vi "Update Controller State.vi"(8 "error in (no error)":errorcluster, 11 "Elevator Controller Actor in":refnum<class "Elevator Controller Actor.lvclass">) -> (0 "error out":errorcluster, 3 "Elevator Controller Actor out":refnum<class "Elevator Controller Actor.lvclass">)   [LabVIEW 2022 SP3, in "Elevator Controller Actor.lvlib" / "Elevator Controller Actor.lvclass"]
uses:
  Elevator Controller Actor.lvclass
  C:/Program Files/National Instruments/LabVIEW 2022/vi.lib/ActorFramework/Actor/Actor.lvclass
  <vilib>/ActorFramework/Actor/Actor.lvclass/Actor.ctl
  <vilib>/ActorFramework/Message Enqueuer/Message Enqueuer.lvclass/Message Enqueuer.ctl
  Elevator Controller Actor.lvclass/Elevator Controller Actor.ctl
  Sim User Console Actor/Elevator Controller Actor/Floor Selection.ctl
  Sim User Console Actor/Elevator Controller Actor/Elevator Call.ctl
  Sim User Console Actor/Elevator Controller Actor/Door Buttons.ctl
  Sim Display Console Actor/Elevator Controller Actor/Elevator Direction.ctl
  Sim Display Console Actor/Elevator Controller Actor/Floor -Enum.ctl
  Configuration Database Actor/Configuration Database Actor/Record -Cluster.ctl
  Configuration Database Actor/Configuration Database Actor Messages/Write Record Msg/Write Record Msg.lvclass/Write Record Msg.ctl
  Sim Sensor Interface Actor/Sim Sensor Interface Actor Messages/Update Elevator Position Msg/Update Elevator Position Msg.lvclass/Update Elevator Position Msg.ctl
  Sim Display Console Actor/Sim Display Console Actor Messages/Update Door Open Msg/Update Door Open Msg.lvclass/Update Door Open Msg.ctl
  Sim Display Console Actor/Sim Display Console Actor Messages/Update Elevator Direction Msg/Update Elevator Direction Msg.lvclass/Update Elevator Direction Msg.ctl
  Sim Display Console Actor/Sim Display Console Actor Messages/Update Elevator Location Msg/Update Elevator Location Msg.lvclass/Update Elevator Location Msg.ctl
  Sim Display Console Actor/Sim Display Console Actor Messages/Update Emergency Msg/Update Emergency Msg.lvclass/Update Emergency Msg.ctl
  Sim Display Console Actor/Sim Display Console Actor Messages/Update Timing Msg/Update Timing Msg.lvclass/Update Timing Msg.ctl
  Sim User Console Actor/Sim User Console Actor Messages/Update Door Buttons Msg/Update Door Buttons Msg.lvclass/Update Door Buttons Msg.ctl
  Sim User Console Actor/Sim User Console Actor Messages/Update Elevator Call Msg/Update Elevator Call Msg.lvclass/Update Elevator Call Msg.ctl
  Sim User Console Actor/Sim User Console Actor Messages/Update Emergency Msg/Update Emergency Msg.lvclass/Update Emergency Msg.ctl
  Sim User Console Actor/Sim User Console Actor Messages/Update Foor Selection Msg/Update Foor Selection Msg.lvclass/Update Foor Selection Msg.ctl
  <vilib>/ActorFramework/Message Enqueuer/Init from Existing Queue.vi
  <vilib>/ActorFramework/Message Enqueuer/Enqueue.vi
  Configuration Database Actor/Configuration Database Actor Messages/Read Record Msg/Read Record Msg.lvclass
  C:/Program Files/National Instruments/LabVIEW 2022/vi.lib/ActorFramework/Message/Message.lvclass
  Configuration Database Actor/Configuration Database Actor Messages/Write Record Msg/Write Record Msg.lvclass
  Sim Sensor Interface Actor/Sim Sensor Interface Actor Messages/Update Elevator Position Msg/Update Elevator Position Msg.lvclass
  Sim Display Console Actor/Sim Display Console Actor Messages/Update Door Open Msg/Update Door Open Msg.lvclass
  Sim Display Console Actor/Sim Display Console Actor Messages/Update Elevator Direction Msg/Update Elevator Direction Msg.lvclass
  Sim Display Console Actor/Sim Display Console Actor Messages/Update Elevator Location Msg/Update Elevator Location Msg.lvclass
  Sim Display Console Actor/Sim Display Console Actor Messages/Update Emergency Msg/Update Emergency Msg.lvclass
  Sim Display Console Actor/Sim Display Console Actor Messages/Update Timing Msg/Update Timing Msg.lvclass
  Sim User Console Actor/Sim User Console Actor Messages/Update Door Buttons Msg/Update Door Buttons Msg.lvclass
  Sim User Console Actor/Sim User Console Actor Messages/Update Elevator Call Msg/Update Elevator Call Msg.lvclass
  Sim User Console Actor/Sim User Console Actor Messages/Update Emergency Msg/Update Emergency Msg.lvclass
  Sim User Console Actor/Sim User Console Actor Messages/Update Foor Selection Msg/Update Foor Selection Msg.lvclass
  Sim User Console Actor/Sim User Console Actor Messages/Read Elevator Call and Floor Selection Msg/Read Elevator Call and Floor Selection Msg.lvclass
  <vilib>/ActorFramework/Message Priority Queue/Priority Enqueue.vi
  <vilib>/ActorFramework/Message Enqueuer/Message Enqueuer.lvclass
  Configuration Database Actor/Configuration Database Actor/Configuration Database Actor.lvclass
  Sim User Console Actor/Elevator Controller Actor/Sim User Console Actor.lvclass
  <vilib>/ActorFramework/Actor/Actor.lvclass
  Sim Display Console Actor/Elevator Controller Actor/Sim Display Console Actor.lvclass
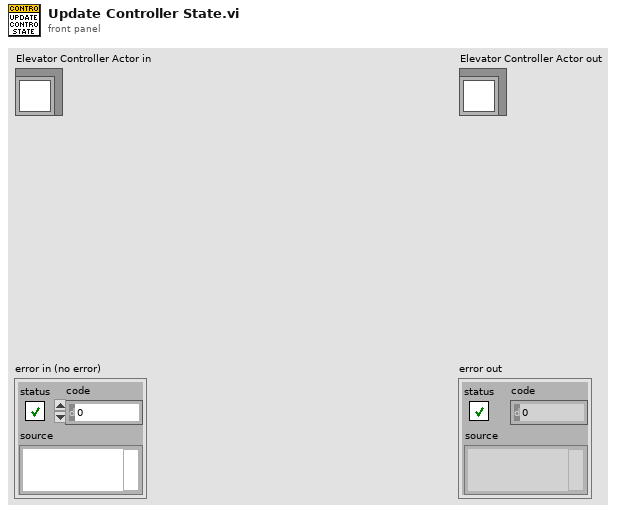
[diagram p1: front panel]
types:
  T1 = typedef "Sim Display Console Actor.lvlib/Sim Display Console Actor.lvclass/Floor -Enum.ctl" = enum16{"1st", "2nd", "3rd", "4th"}
  T2 = typedef "Sim Display Console Actor.lvlib/Sim Display Console Actor.lvclass/Elevator Direction.ctl" = cluster{"Up":bool, "Down":bool}
  T3 = typedef "Sim User Console Actor.lvlib/Sim User Console Actor.lvclass/Door Buttons.ctl" = cluster{"Open Door":bool, "Close Door":bool}
  T4 = typedef "Sim User Console Actor.lvlib/Sim User Console Actor.lvclass/Elevator Call.ctl" = cluster{"Up":bool, "Up 2":bool, "Up 3":bool, "Down":bool, "Down 2":bool, "Down 3":bool}
  T5 = typedef "Sim User Console Actor.lvlib/Sim User Console Actor.lvclass/Floor Selection.ctl" = cluster{"Floor4":bool, "Floor 3":bool, "Floor2":bool, "Floor1":bool}
  T6 = typedef "Configuration Database Actor.lvlib/Configuration Database Actor.lvclass/Record -Cluster.ctl" = cluster{"Door Open":dbl, "Door Close":dbl, "Travel Time":dbl, "Inactivity Time":dbl}
  T7 = typedef "Elevator Controller Actor.lvlib/Elevator Controller Actor.lvclass/State -Enum.ctl" = enum16{"Initial", "Wait for First Request", "Start and Move", "Anaysis", "Continue Travel", "Stop at Floor", "Open and Close Door Sequence", "No Request Remaining", "Emergency Call", "Terminate Process"}
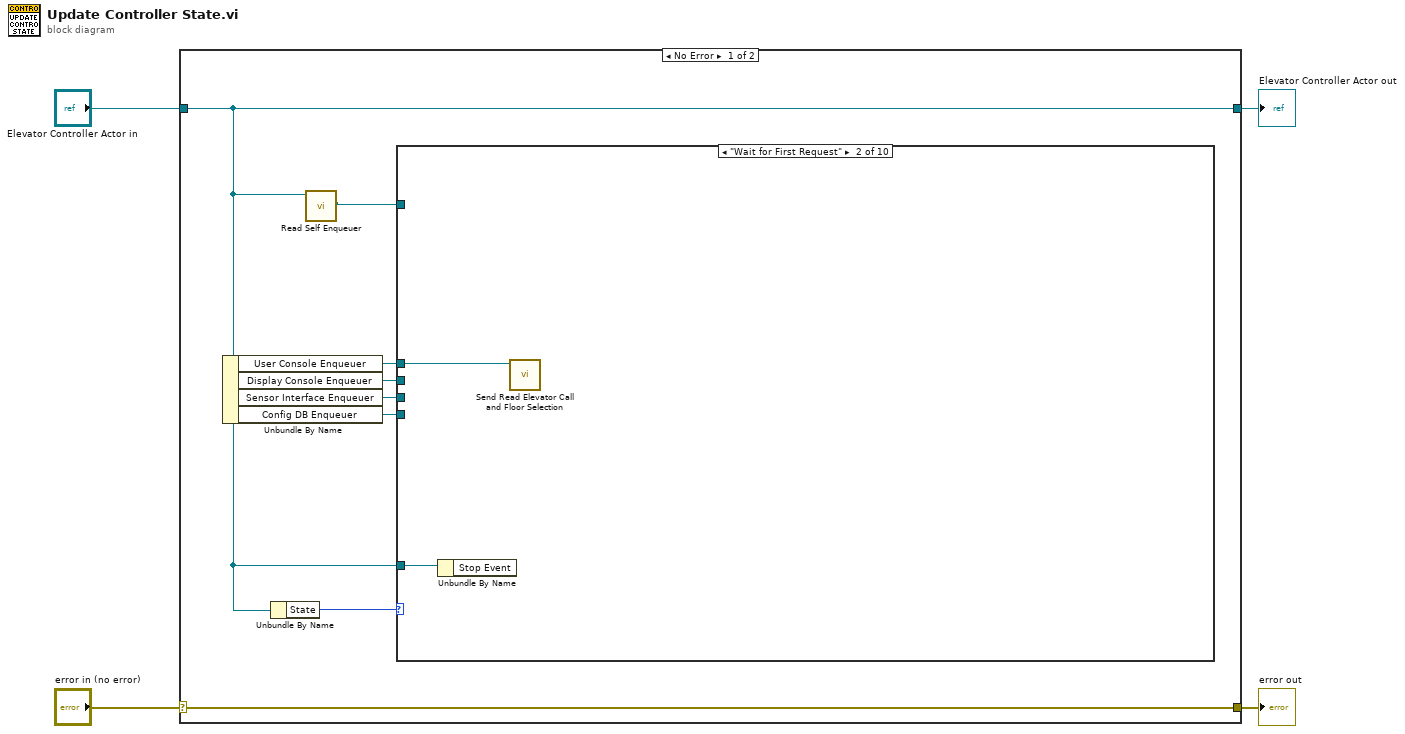
[diagram p0: block diagram]
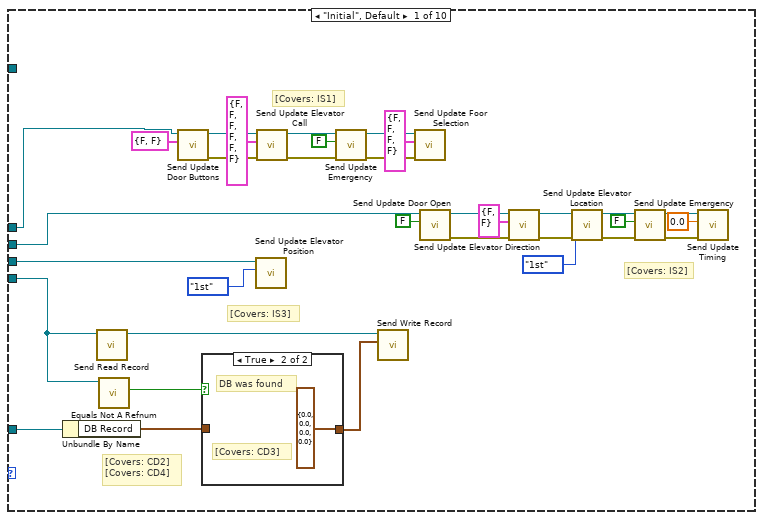
[diagram p2: hidden frame]
diagram:
  n1 = case shown="No Error" "error in (no error)" {
    selector: "error in (no error)" -> [w12 w51]
    tunnel: [w12 w51] -> w3
    tunnel: [w6 w50] -> w1
    tunnel: "Elevator Controller Actor in" -> [w6 w50]
    frame No Error {
      n2 = Unbundle By Name(w6) -> ("User Console Enqueuer"=w10:refnum<class "Message Enqueuer.lvclass">, "Display Console Enqueuer"=w9:refnum<class "Message Enqueuer.lvclass">, "Sensor Interface Enqueuer"=w8:refnum<class "Message Enqueuer.lvclass">, "Config DB Enqueuer"=w7:refnum<class "Message Enqueuer.lvclass">)
      n3 = Unbundle By Name(w6) -> ("State"=w11:T7)
      n4 = call <vilib>:"Read Self Enqueuer.vi"("Actor"=w6) -> ("Self Enqueuer"=w5:refnum<class "Message Enqueuer.lvclass">)  [unwired: 10 in]
      n5 = case shown="\"Wait for First Request\"" w11 {
        tunnel: w10 -> [w29 w49 _ _ _ _ _ _ _ _]
        tunnel: w9 -> [w20 _ _ _ _ _ _ _ _ _]
        tunnel: w8 -> [w14 _ _ _ _ _ _ _ _ _]
        tunnel: w7 -> [w43 _ _ _ _ _ _ _ _ _]
        tunnel: w6 -> [w44 w48 _ _ _ _ _ _ _ _]
        tunnel: w5 -> [_ _ _ _ _ _ _ _ _ _]
        frame "Initial", Default {
          # "[Covers: IS3]"
          # "[Covers: IS2]"
          # "[Covers: IS1]"
          # "[Covers: CD2] \n[Covers: CD4]"
          n6 = Unbundle By Name(w44) -> ("DB Record"=w41:T6)
          n7 = call "Send Read Record.vi"("Message Enqueuer"=w43) -> ("Message Enqueuer out"=w45:refnum<class "Message Enqueuer.lvclass">)  [unwired: 9 in, 1 out]
          n8 = call <vilib>:"Equals Not A Refnum.vi"("Message Enqueuer"=w43) -> ("Not a refnum?"=w42:bool)  [unwired: 10 in]
          n9 = call "Send Update Door Buttons.vi"("Door Buttons"=T3 {"Open Door"=FALSE, "Close Door"=FALSE}, "Message Enqueuer"=w29) -> ("error out"=w39:errorcluster, "Message Enqueuer out"=w36:refnum<class "Message Enqueuer.lvclass">)  [unwired: 8 in]
          n10 = case shown="True" w42 {
            tunnel: w41 -> [w46 _]
            tunnel: [w46 T6 {"Door Open"=0.0, "Door Close"=0.0, "Travel Time"=0.0, "Inactivity Time"=0.0} ("DB Record")] -> w40
            frame False {
            }
            frame True {
              # "[Covers: CD3]"
              # "DB was found"
            }
          }
          n11 = call "Send Update Elevator Position.vi"("Elevator Position"=Floor_-Enum."1st" ("Elevator Location"), "Message Enqueuer"=w14) -> ()  [unwired: 8 in, 2 out]
          n12 = call "Send Update Elevator Call.vi"("error in (no error)"=w39, "Elevator call"=T4 {"Up"=FALSE, "Up 2"=FALSE, "Up 3"=FALSE, "Down"=FALSE, "Down 2"=FALSE, "Down 3"=FALSE}, "Message Enqueuer"=w36) -> ("error out"=w38:errorcluster, "Message Enqueuer out"=w35:refnum<class "Message Enqueuer.lvclass">)  [unwired: 7 in]
          n13 = call "Send Update Emergency.vi"("error in (no error)"=w38, "Emergency"=FALSE, "Message Enqueuer"=w35) -> ("error out"=w37:errorcluster, "Message Enqueuer out"=w34:refnum<class "Message Enqueuer.lvclass">)  [unwired: 7 in]
          n14 = call "Send Write Record.vi"("Record"=w40, "Message Enqueuer"=w45) -> ()  [unwired: 8 in, 2 out]
          n15 = call "Send Update Foor Selection.vi"("error in (no error)"=w37, "Floor Selection"=T5 {"Floor4"=FALSE, "Floor 3"=FALSE, "Floor2"=FALSE, "Floor1"=FALSE}, "Message Enqueuer"=w34) -> ()  [unwired: 7 in, 2 out]
          n16 = call "Send Update Door Open.vi"("Door Open"=FALSE, "Message Enqueuer"=w20) -> ("error out"=w28:errorcluster, "Message Enqueuer out"=w24:refnum<class "Message Enqueuer.lvclass">)  [unwired: 8 in]
          n17 = call "Send Update Elevator Direction.vi"("error in (no error)"=w28, "Elevator Direction"=T2 {"Up"=FALSE, "Down"=FALSE}, "Message Enqueuer"=w24) -> ("error out"=w27:errorcluster, "Message Enqueuer out"=w23:refnum<class "Message Enqueuer.lvclass">)  [unwired: 7 in]
          n18 = call "Send Update Elevator Location.vi"("error in (no error)"=w27, "Elevator Location"=Floor_-Enum."1st", "Message Enqueuer"=w23) -> ("error out"=w26:errorcluster, "Message Enqueuer out"=w22:refnum<class "Message Enqueuer.lvclass">)  [unwired: 7 in]
          n19 = call "Send Update Emergency.vi"("error in (no error)"=w26, "Emergency"=FALSE, "Message Enqueuer"=w22) -> ("error out"=w25:errorcluster, "Message Enqueuer out"=w21:refnum<class "Message Enqueuer.lvclass">)  [unwired: 7 in]
          n20 = call "Send Update Timing.vi"("error in (no error)"=w25, "Timing"=0.0, "Message Enqueuer"=w21) -> ()  [unwired: 7 in, 2 out]
        }
        frame "Wait for First Request" {
          n21 = Unbundle By Name(w48) -> ()  [unwired: 1 out]
          n22 = call "Send Read Elevator Call and Floor Selection.vi"("Message Enqueuer"=w49) -> ()  [unwired: 9 in, 2 out]
        }
        frame "Start and Move" {
        }
        frame "Anaysis" {
        }
        frame "Continue Travel" {
        }
        frame "Stop at Floor" {
        }
        frame "Open and Close Door Sequence" {
        }
        frame "No Request Remaining" {
        }
        frame "Emergency Call" {
        }
        frame "Terminate Process" {
        }
      }
    }
    frame Error {
    }
  }
  "error out" <- w3
  "Elevator Controller Actor out" <- w1
